vi "FactorialOperations.vi"(0 "M":i32, 5 "N":i32, 7 "Operations":T1, 9 "?":bool) -> (4 "C":u64)   [LabVIEW 2020]
doc: "This VI performs factorial based operations on the two numbers M and N as per user input"
uses:
  Typedefs/Operations.ctl
panel:
  # "This program performs operations on the numbers M and N as per user input."
  # "INPUT"
  # "OUTPUT"
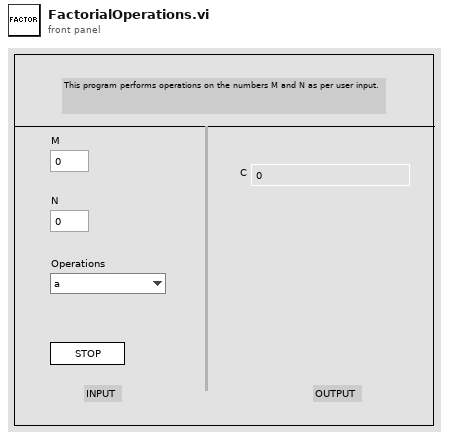
[diagram p1: front panel]
types:
  T1 = typedef "Operations.ctl" = enum16{"a", "b", "c", "d"}
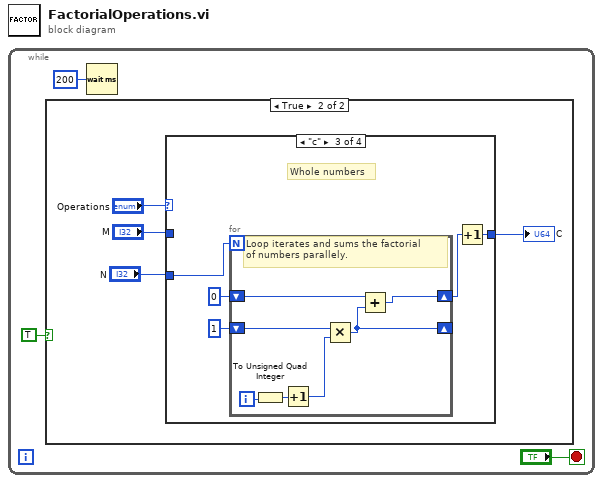
[diagram p0: block diagram]
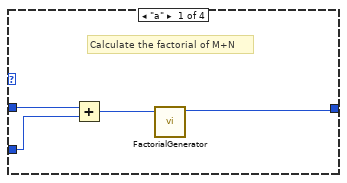
[diagram p3: hidden frame]
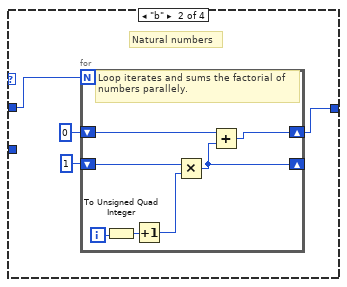
[diagram p4: hidden frame]
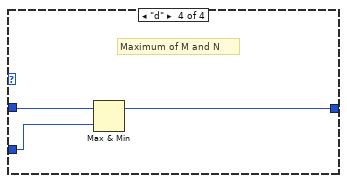
[diagram p5: hidden frame]
diagram:
  n1 = while {
    stop <- "?" stop-if-true
    n2 = case shown="True" TRUE {
      frame False {
      }
      frame True {
        n3 = case shown="\"c\"" "Operations" {
          tunnel: "M" -> [w11 w13 _ w37]
          tunnel: "N" -> [w10 _ w25 w36]
          tunnel: [w8 w12 w24 w35] -> w4
          frame "a" {
            # "Calculate the factorial of M+N"
            n4 = Add(x=w11, y=w10) -> (x+y=w9:i32)
            n5 = call "FactorialGenerator.vi"("Numeric"=w9) -> ("Numeric 2"=w8:u64)  [unwired: 10 in]
          }
          frame "b" {
            # "Natural numbers"
            n6 = for {
              N: w13 -> [_]
              shift-right: [w17] -> w12
              shift-left: 0 -> [w16]
              shift-right: [w21] -> _
              shift-left: 1 -> [w22]
              i -> [w18]
              # "Loop iterates and sums the factorial of numbers parallely."
              n7 = To Unsigned Quad Integer(1:w18) -> (0:w19:u64)
              n8 = Increment(x=w19) -> (x+1=w20:u64)
              n9 = Multiply(x=w22, y=w20) -> (x*y=w21:u64)
              n10 = Add(x=w16, y=w21) -> (x+y=w17:u64)
            }
          }
          frame "c" {
            # "Whole numbers"
            n11 = for {
              N: w25 -> [_]
              shift-right: [w29] -> w23
              shift-left: u64 0 -> [w28]
              shift-right: [w33] -> _
              shift-left: u64 1 -> [w34]
              i -> [w30]
              # "Loop iterates and sums the factorial \nof numbers parallely."
              n12 = To Unsigned Quad Integer(1:w30) -> (0:w31:u64)
              n13 = Increment(x=w31) -> (x+1=w32:u64)
              n14 = Multiply(x=w34, y=w32) -> (x*y=w33:u64)
              n15 = Add(x=w28, y=w33) -> (x+y=w29:u64)
            }
            n16 = Increment(x=w23) -> (x+1=w24:u64)
          }
          frame "d" {
            # "Maximum of M and N"
            n17 = Max & Min(x=w37, y=w36) -> (max(x,y)=w35:i32)  [unwired: 1 out]
          }
        }
        "C" <- w4
      }
    }
    n18 = Wait (ms)(milliseconds to wait=u32 200) -> ()  [unwired: 1 out]
  }
